vi "Send Read Single-Point.vi"(7 "Message Priority (Normal)":T1=enum."Normal", 8 "error in (no error)":errorcluster, 10 "maximum time (5s)":dbl[unit]=5000.0 caption="maximum time (5000 ms)", 11 "Message Enqueuer":refnum<class "Message Enqueuer.lvclass">) -> (0 "error out":errorcluster, 3 "Message Enqueuer out":refnum<class "Message Enqueuer.lvclass">)   [LabVIEW 2015, in "CS++DMM.lvlib" / "Read Single-Point Msg.lvclass"]
doc: "Sends the <B>CS++DMM.lvlib:Read Single-Point Msg.lvclass</B> message.\n\n<B>CS++DMM.lvlib:CS++DMM.lvclass:Read Single-Point.vi</B> Description:\n\nThis VI initiates a measurement, waits until the DMM has returned to the Idle state, and returns the measured value.\n\nThis VI applies default values to properties that have not been set by the user under the following conditions:\n\n(1) If the user has not set the value of any property in the IviDmmMultiPoint extension group, the VI sets the IviDmm>>Multi-Point Acquisition>>Sample Count [MP] and IviDmm>>Multi-Point Acquisition>>Trigger Count [MP] properties to 1.\n\n(2) If the user has not set the value of the IviDmm>Measurement Operation Options>Auto Zero [AZ] property, the VI sets the value of this property to IVIDMM_VAL_AUTO_ZERO_OFF (0). \n\nNotes:\n\n(1) After this VI executes, the Reading parameter contains an actual reading or a value indicating that an over-range condition occurred.\n\n(2) If an over-range condition occurs, the Reading parameter contains an IEEE defined NaN (Not a Number) value and the VI returns the IVIDMM_WARN_OVER_RANGE (0x3ffA2001) warning code.\n\n(3) You can test the measurement value for an over-range condition by calling the IviDmm Is Over-Range VI.\n\n(4) This VI performs interchangeability checking when the IviDmm>>Inherent IVI Settings>>User Options>>Interchange Check property is set to TRUE. If the IviDmm>>Inherent IVI Settings>>User Options>>Spy property is set to TRUE, you use the NI Spy utility to view interchangeability warnings. You use the IviDmm Get Next Interchange Warning VI to retrieve interchangeability warnings when the IviDmm>>Inherent IVI Settings>>User Options>>Spy property is set to FALSE. For more information about interchangeability checking, refer to the help text for the IviDmm>>Inherent IVI Settings>>User Options>>Interchange Check property.\n\n(5) The class driver returns a simulated measurement when this VI is called and the IviDmm>>Inherent IVI Settings>>User Options>>Simulate property is set to TRUE and the IviDmm>>Inherent IVI Settings>>User Options>>Use Specific Simulation property is set to FALSE. For information on how to configure a simulated measurement, refer to the online help manual."
uses:
  Read Single-Point Msg.lvclass
  <vilib>/ActorFramework/Message Enqueuer/Message Enqueuer.lvclass
  <vilib>/ActorFramework/Message Enqueuer/Message Priority.ctl
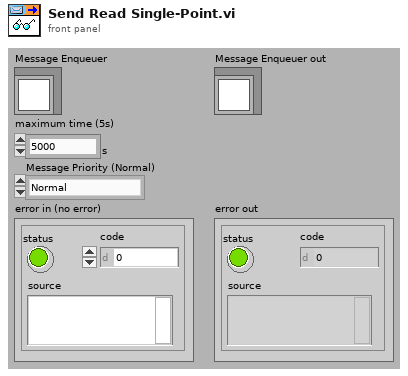
[diagram p1: front panel]
types:
  T1 = typedef "Actor Framework.lvlib/Message Enqueuer.lvclass/Message Priority.ctl" = enum16{"Low", "Normal", "High"}
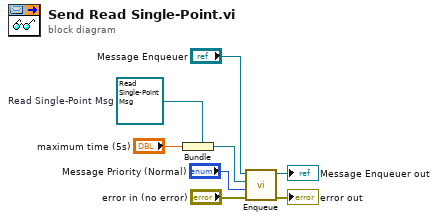
[diagram p0: block diagram]
diagram:
  w2 = refnum<class "Read Single-Point Msg.lvclass"> refnum  # Read Single-Point Msg
  n1 = Bundle(cluster=w2, "maximum time (5s)") -> (w5:refnum<class "Read Single-Point Msg.lvclass">)
  n2 = call <vilib>:"Enqueue.vi"("error in (no error)"="error in (no error)", "Message Priority (Normal)"="Message Priority (Normal)", "Message"=w5, "Message Enqueuer in"="Message Enqueuer") -> ("error out"=→"error out":errorcluster, "Message Enqueuer out"=→"Message Enqueuer out":refnum<class "Message Enqueuer.lvclass">)  [unwired: 6 in]
